vi "Write.vi"(8 "ErrorIn":errorcluster, 10 "Command":string, 11 "VISAIn":refnum<visa-resource-name>) -> (0 "ErrorOut":errorcluster, 3 "VISAOut":refnum<visa-resource-name>)   [LabVIEW 2017, in "I28Drivers.lvlib"]
uses:
  I28Drivers.lvlib
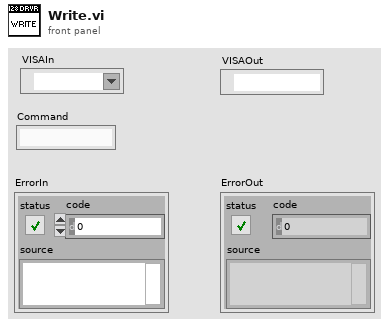
[diagram p1: front panel]
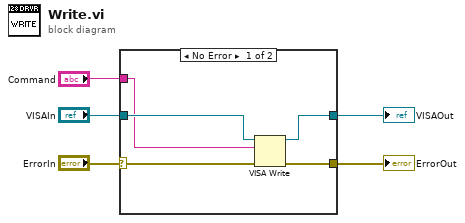
[diagram p0: block diagram]
diagram:
  n1 = case shown="No Error" "ErrorIn" {
    selector: "ErrorIn" -> [w6 w11]
    tunnel: [w7 w11] -> w4
    tunnel: "VISAIn" -> [w10 w12]
    tunnel: "Command" -> [w8 _]
    tunnel: [w9 w12] -> w1
    frame No Error {
      n2 = VISA Write(VISA resource name=w10, write buffer=w8, error in (no error)=w6) -> (VISA resource name out=w9:refnum<visa-resource-name>, error out=w7:errorcluster)  [unwired: 1 out]
    }
    frame Error {
    }
  }
  "ErrorOut" <- w4
  "VISAOut" <- w1
